vi "Hypo-T.vi"(3 "How?Forebrain":cluster{"Motor1":i16, "Motor 2":i16}) -> (1 "Act Out":cluster{"Motor1":i16, "Motor 2":i16})   [LabVIEW 2012]
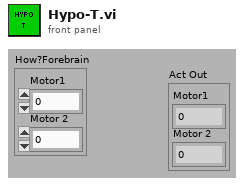
[diagram p1: front panel]
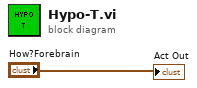
[diagram p0: block diagram]
diagram:
  "Act Out" <- "How?Forebrain"
